vi "CSC_GetCableJacobian.vi"(8 "error in (no error)":errorcluster, 11 "C-Alex in":refnum<class "CableSerialChain.lvclass">) -> (0 "error out":errorcluster, 2 "Jacobian for Cables":T1, 3 "C-Alex out":refnum<class "CableSerialChain.lvclass">)   [LabVIEW 2015, in "CableSerialChain.lvclass"]
uses:
  CableSerialChain.lvclass
  <vilib>/Analysis/Matrix/Datatypes/RealMatrix.ctl
  CableSerialChain.lvclass/CableSerialChain.ctl
  Body/Force.ctl
  Body/PointOnBody.ctl
  <vilib>/Analysis/BLAS.llb/dnrm2 - Vector 2-Norm (DBL).vi
  <vilib>/Analysis/Matrix/Numeric/Conversions/Array To Matrix - RA2.vi
  Body/Bodies.lvclass
  <vilib>/Analysis/NI_AALBLAS.lvlib
  <vilib>/Analysis/Matrix/NI_Matrix.lvlib
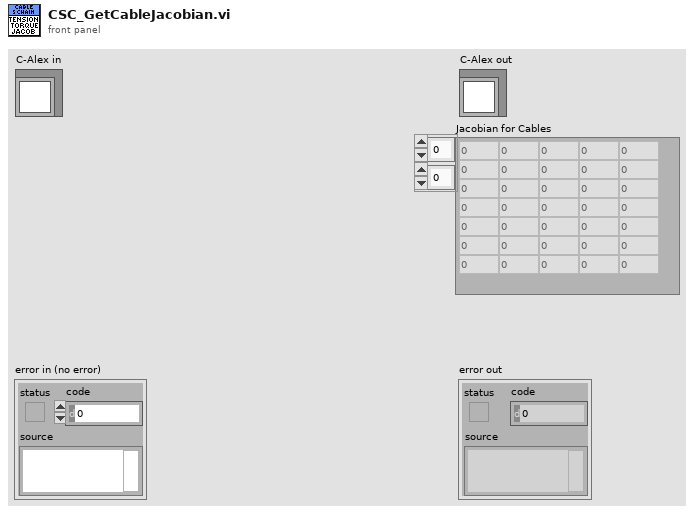
[diagram p1: front panel]
types:
  T1 = typedef "NI_Matrix.lvlib/RealMatrix.ctl" = dbl[][]
  T2 = typedef "Bodies.lvclass/Force.ctl" = cluster{"LocationInLCS":T3, "ForceVector":dbl[]}
  T3 = typedef "Bodies.lvclass/PointOnBody.ctl" = cluster{"Coord4":dbl[], "ID":i32}
  T4 = typedef "CableSerialChain.lvclass/Cable.ctl" = cluster{"RoutingPtsInLCS":T3[], "Cable ID":i32, "ActiveSegments":i32[][]}
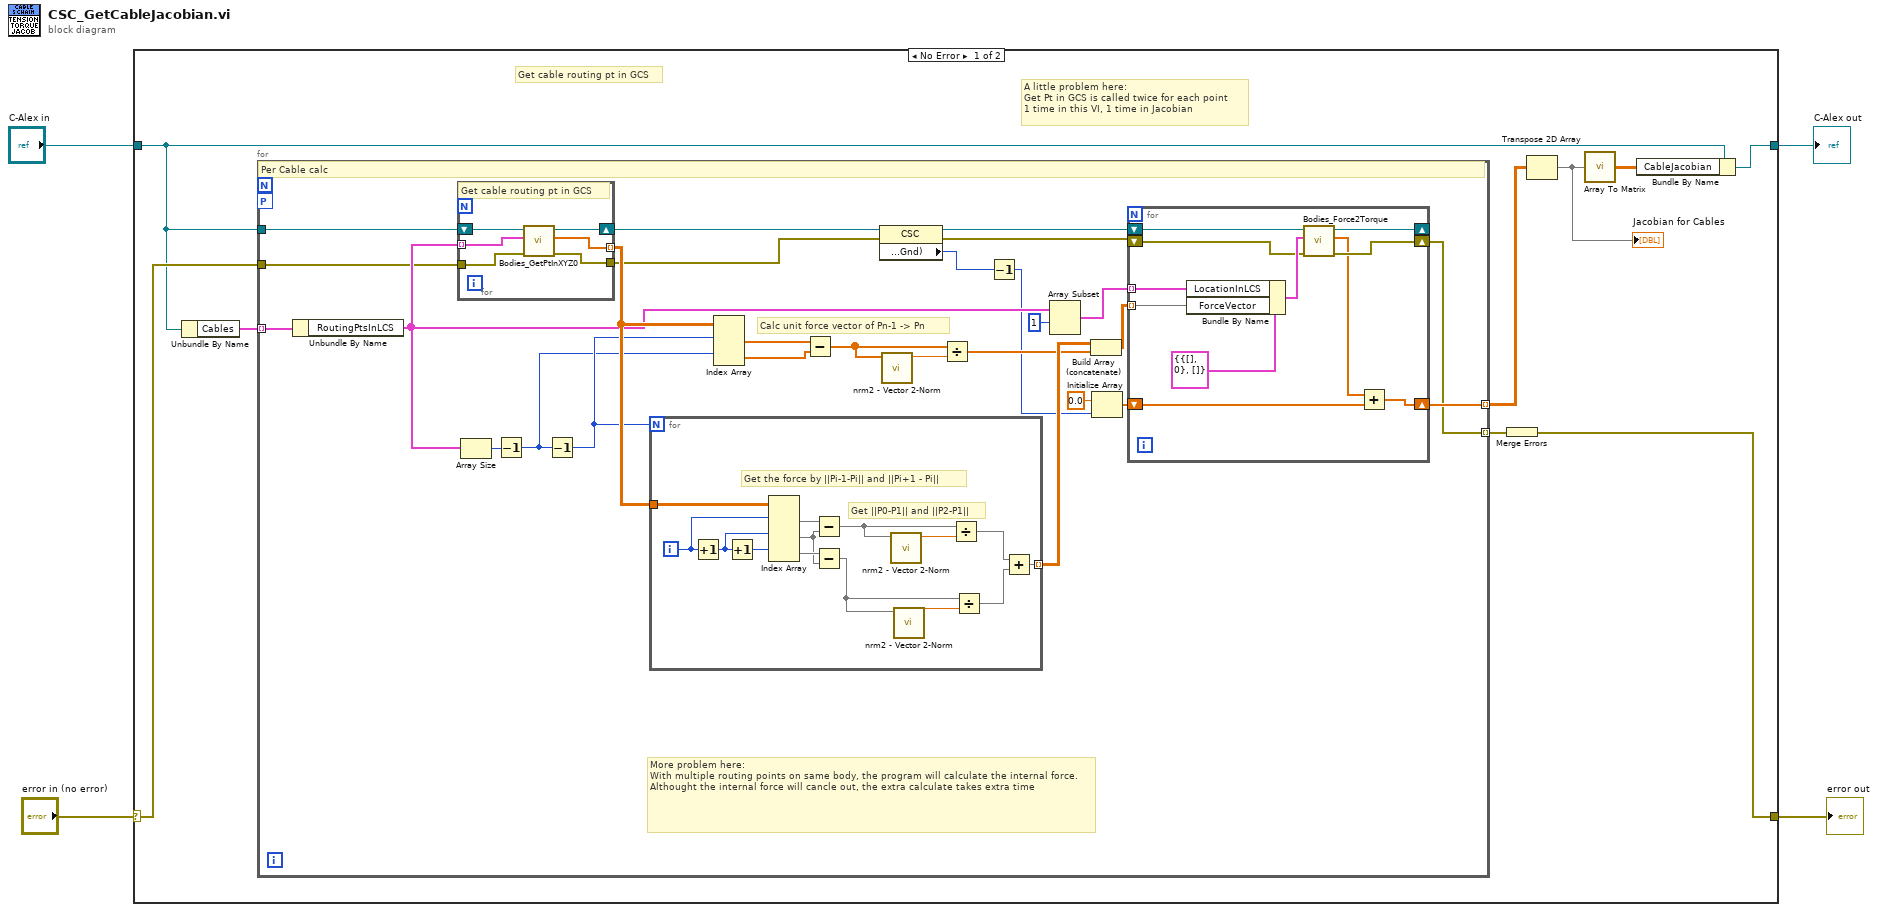
[diagram p0: block diagram]
diagram:
  n1 = case shown="No Error" "error in (no error)" {
    selector: "error in (no error)" -> [w12 w72]
    tunnel: [w8 w72] -> w3
    tunnel: [w7 w73] -> w1
    tunnel: "C-Alex in" -> [w5 w73]
    frame No Error {
      # "Get cable routing pt in GCS"
      # "A little problem here:\nGet Pt in GCS is called twice for each point\n1 time in this VI, 1 time in Jacobian"
      n2 = Unbundle By Name(w5) -> ("Cables"=w13:T4[])
      n3 = for {
        tunnel: w13 -> [w40] mode=indexing
        tunnel: [w25] -> w10 mode=indexing
        workers-P: _ -> [_]
        tunnel: w12 -> [w15]
        tunnel: [w14] -> w11 mode=indexing
        tunnel: w5 -> [w39]
        # "More problem here:\nWith multiple routing points on same body, the program will calculate the internal force. Althought the internal force will cancle out, the extra calculate takes extra time"
        # "Calc unit force vector of Pn-1 -> Pn"
        # "Per Cable calc"
        n4 = Unbundle By Name(w40) -> ("RoutingPtsInLCS"=w28:T3[])
        n5 = for {
          tunnel: w28 -> [w55] mode=indexing
          shift-right: [w56] -> w21
          shift-left: w39 -> [w57]
          tunnel: w15 -> [w54]
          tunnel: [w53] -> w19
          tunnel: [w52] -> w38 mode=indexing
          # "Get cable routing pt in GCS"
          n6 = call "Bodies_GetPtInXYZ0.vi"("error in (no error)"=w54, "Point"=w55, "Bodies.lvclass"=w57) -> ("error out"=w53:errorcluster, "PointInGCS"=w52:dbl[], "Bodies.lvclass 2"=w56:refnum<class "CableSerialChain.lvclass">)  [unwired: 5 in, 1 out]
        }
        n7 = Array Size(array=w28) -> (size(s)=w37:i32)
        n8 = Decrement(x=w37) -> (x-1=w22:i32)
        n9 = Decrement(x=w22) -> (x-1=w36:i32)
        n10 = for {
          N: w36 -> [_]
          tunnel: w38 -> [w71]
          tunnel: [w58] -> w31 mode=indexing
          i -> [w70]
          # "Get the force by ||Pi-1-Pi|| and ||Pi+1 - Pi||"
          # "Get ||P0-P1|| and ||P2-P1||"
          n11 = Increment(x=w70) -> (x+1=w69:i32)
          n12 = Increment(x=w69) -> (x+1=w68:i32)
          n13 = Index Array(array=w71, index (row) #1=w70, index (row) #2=w69, index (row) #3=w68) -> (element #1=w67:dbl[], element #2=w65:dbl[], element #3=w66:dbl[])  [unwired: 3 in]
          n14 = Subtract(x=w67, y=w65) -> (x-y=w64:dbl[])
          n15 = Subtract(x=w66, y=w65) -> (x-y=w61:dbl[])
          n16 = call-poly <vilib>:"nrm2 - Vector 2-Norm.vi"("x"=w64) -> ("dnrm2"=w63:dbl)  [unwired: 9 in, 1 out]
          n17 = call-poly <vilib>:"nrm2 - Vector 2-Norm.vi"("x"=w61) -> ("dnrm2"=w62:dbl)  [unwired: 9 in, 1 out]
          n18 = Divide(x=w64, y=w63) -> (x/y=w60:dbl[])
          n19 = Divide(x=w61, y=w62) -> (x/y=w59:dbl[])
          n20 = Add(x=w60, y=w59) -> (x+y=w58:dbl[])
        }
        n21 = Index Array(array=w38, index (row) #1=w36, index (row) #2=w22) -> (element #1=w33:dbl[], element #2=w32:dbl[])  [unwired: 2 in]
        n22 = Subtract(x=w33, y=w32) -> (x-y=w34:dbl[])
        n23 = property class="CSC"(reference=w21, error in=w19) -> (reference out=w20:refnum<class "CableSerialChain.lvclass">, error out=w18:errorcluster, "#ofBodies(Inc.Gnd)"=w17:i32)
        n24 = call-poly <vilib>:"nrm2 - Vector 2-Norm.vi"("x"=w34) -> ("dnrm2"=w35:dbl)  [unwired: 9 in, 1 out]
        n25 = Divide(x=w34, y=w35) -> (x/y=w30:dbl[])
        n26 = Decrement(x=w17) -> (x-1=w16:i32)
        n27 = Array Subset(array=w28, index=1) -> (w26:T3[])  [unwired: 1 in]
        n28 = Build Array (concatenate)(w31, w30) -> (w29:dbl[][])
        n29 = Initialize Array(0.0 ("element"), w16) -> (w24:dbl[])
        n30 = for {
          tunnel: w29 -> [w50] mode=indexing
          tunnel: w26 -> [w45] mode=indexing
          shift-right: [w44] -> w14
          shift-left: w18 -> [w47]
          shift-right: [w46] -> _
          shift-left: w20 -> [w49]
          shift-right: [w42] -> w25
          shift-left: w24 -> [w41]
          n31 = Bundle By Name(cluster=T2 {"LocationInLCS"={"Coord4"=[], "ID"=0}, "ForceVector"=[]} ("Force"), "LocationInLCS"=w45, "ForceVector"=w50) -> (w48:T2)
          n32 = call "Bodies_Force2Torque.vi"("error in (no error)"=w47, "Force"=w48, "Bodies.lvclass"=w49) -> ("error out"=w44:errorcluster, "Torque Vector"=w43:dbl[], "Bodies.lvclass 2"=w46:refnum<class "CableSerialChain.lvclass">)  [unwired: 5 in, 1 out]
          n33 = Add(x=w43, y=w41) -> (x+y=w42:dbl[])
        }
      }
      n34 = Merge Errors(w11) -> (w8:errorcluster)
      n35 = Transpose 2D Array(2D array=w10) -> (transposed array=w9:dbl[][])
      "Jacobian for Cables" <- w9
      n36 = call-poly <vilib>:"Array To Matrix.vi"("Real 2D Array"=w9) -> ("Real Matrix"=w6:T1)
      n37 = Bundle By Name(cluster=w5, "CableJacobian"=w6) -> (w7:refnum<class "CableSerialChain.lvclass">)
    }
    frame Error {
    }
  }
  "error out" <- w3
  "C-Alex out" <- w1
